vi "Menu-Stop Imp.vi"(8 "error in":errorcluster, 11 "Menu in":refnum<k9>) -> ()   [LabVIEW 2016, in "CML UI.lvlib"]
uses:
  CML UI.lvlib
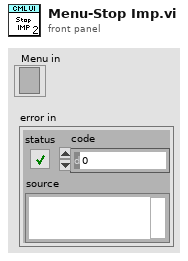
[diagram p1: front panel]
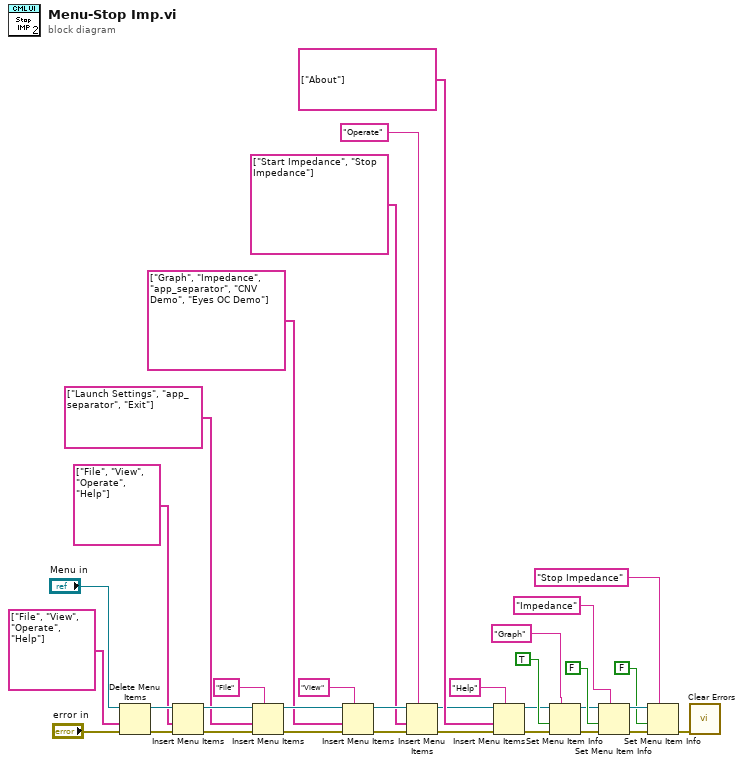
[diagram p0: block diagram]
diagram:
  n1 = Delete Menu Items(6:"error in", 7:string[] ["File", "View", "Operate", "Help"] ("L10n_item tags 1"), 9:"Menu in") -> (0:w35:errorcluster, 3:w34:refnum<k9>)  [unwired: 1 in]
  n2 = Insert Menu Items(6:w35, 7:string[] ["File", "View", "Operate", "Help"] ("L10n_item tags 1"), 9:w34) -> (0:w21:errorcluster, 3:w23:refnum<k9>)  [unwired: 3 in, 1 out]
  n3 = Insert Menu Items(5:"File" ("L10n_menu tag"), 6:w21, 7:string[] ["Launch Settings", "app_separator", "Exit"] ("L10n_item tags 2"), 9:w23) -> (0:w16:errorcluster, 3:w17:refnum<k9>)  [unwired: 2 in, 1 out]
  n4 = Insert Menu Items(5:"View" ("L10n_menu tag"), 6:w16, 7:string[] ["Graph", "Impedance", "app_separator", "CNV Demo", "Eyes OC Demo"] ("L10n_item tags 2"), 9:w17) -> (0:w12:errorcluster, 3:w13:refnum<k9>)  [unwired: 2 in, 1 out]
  n5 = Insert Menu Items(5:"Operate" ("L10n_menu tag"), 6:w12, 7:string[] ["Start Impedance", "Stop Impedance"] ("L10n_item tags 2"), 9:w13) -> (0:w26:errorcluster, 3:w25:refnum<k9>)  [unwired: 2 in, 1 out]
  n6 = Insert Menu Items(5:"Help" ("L10n_menu tag"), 6:w26, 7:string[] ["About"] ("L10n_item tags 2"), 9:w25) -> (0:w2:errorcluster, 3:w5:refnum<k9>)  [unwired: 2 in, 1 out]
  n7 = Set Menu Item Info(7:"Graph" ("item tag"), 8:w2, 9:TRUE ("enabled"), 11:w5) -> (0:w3:errorcluster, 3:w4:refnum<k9>)  [unwired: 3 in]
  n8 = Set Menu Item Info(7:"Impedance" ("item tag"), 8:w3, 9:FALSE ("enabled"), 11:w4) -> (0:w33:errorcluster, 3:w32:refnum<k9>)  [unwired: 3 in]
  n9 = Set Menu Item Info(7:"Stop Impedance" ("item tag"), 8:w33, 9:FALSE ("enabled"), 11:w32) -> (0:w7:errorcluster)  [unwired: 3 in, 1 out]
  n10 = call <vilib>:"Clear Errors.vi"("error in (no error)"=w7) -> ()  [unwired: 5 in, 2 out]
